vi "rotate.vi"(0 "Angle":dbl, 1 "Rate":dbl=-4.0) -> (2 "finished?":bool, 3 "left speed":dbl, 4 "right speed":dbl)   [LabVIEW 2012]
doc: "Rotates the robot for a certain number of degrees at a certain rate."
uses:
  <vilib>/addons/control/pid/pid.llb/PID Control Input Filter (DBL).vi
  <vilib>/addons/control/pid/NI_PID_pid.lvlib
  <vilib>/addons/control/pid/pid.llb/PID (DBL).vi
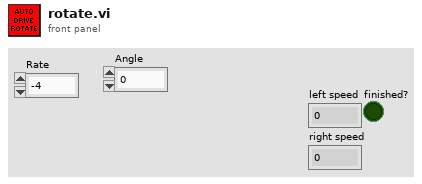
[diagram p1: front panel]
types:
  T1 = typedef "subStates.ctl" = enum16{"null", "wait", "driver control", "auto", "manual override", "hold position", "rotate", "feeder", "end"}
  T2 = typedef "WPI_EncoderDevRef.ctl" = cluster{"DevStatus":errorcluster, "EncoderIndex":T3, "CounterIndex":T4, "DistancePerCount":dbl, "Decoding Type":T5}
  T3 = typedef "FPGA_EncoderIdx.ctl" = enum8{"Enc 0", "Enc 1", "Enc 2", "Enc 3", "Invalid"}
  T4 = typedef "FPGA_CounterCtrSystemIndex.ctl" = enum8{"Ctr 0", "Ctr 1", "Ctr 2", "Ctr 3", "Ctr 4", "Ctr 5", "Ctr 6", "Ctr 7", "Invalid"}
  T5 = typedef "WPI_EncoderType.ctl" = enum16{"1x", "2x", "4x"}
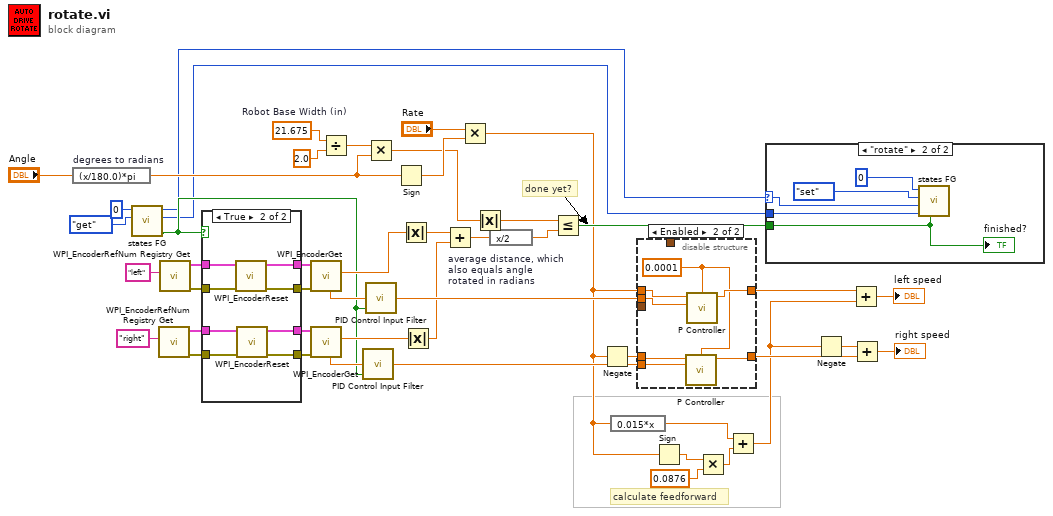
[diagram p0: block diagram]
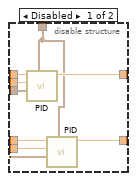
[diagram p2: hidden frame]
diagram:
  w46 = 21.675  # Robot Base Width (in)
  # "calculate feedforward"
  # "done yet?"
  n1 = expression code="(x/180.0)*pi" "degrees to radians"("Angle") -> (w4:dbl)
  n2 = call "states FG.vi"("menu (get)"=enum16{"set", "get"}."get", "Loop ID"=0) -> ("first call?"=w19:bool, "state # out"=w2:i32, "subState out"=w1:T1)  [unwired: 6 in, 1 out]
  n3 = call <vilib>:"WPI_EncoderRefNum Registry Get.vi"("refnum name"="right") -> ("error out"=w30:errorcluster, "EncoderDevRef"=w31:T2)  [unwired: 9 in]
  n4 = call <vilib>:"WPI_EncoderRefNum Registry Get.vi"("refnum name"="left") -> ("error out"=w32:errorcluster, "EncoderDevRef"=w33:T2)  [unwired: 9 in]
  n5 = case shown="True" w19 {
    tunnel: w33 -> [w51 w57]
    tunnel: w32 -> [w50 w59]
    tunnel: w31 -> [w49 w54]
    tunnel: w30 -> [w48 w55]
    tunnel: [w50 w58] -> w29
    tunnel: [w51 w56] -> w28
    tunnel: [w49 w53] -> w27
    tunnel: [w48 w52] -> w26
    frame False {
    }
    frame True {
      n6 = call <vilib>:"WPI_EncoderReset.vi"("error in (no error)"=w59, "EncoderDevRef"=w57) -> ("error out"=w58:errorcluster, "EncoderDevRef"=w56:T2)  [unwired: 8 in]
      n7 = call <vilib>:"WPI_EncoderReset.vi"("error in (no error)"=w55, "EncoderDevRef"=w54) -> ("error out"=w52:errorcluster, "EncoderDevRef"=w53:T2)  [unwired: 8 in]
    }
  }
  n8 = call <vilib>:"WPI_EncoderGet.vi"("error in (no error)"=w29, "EncoderDevRef"=w28) -> ("Distance"=w25:dbl, "Rate"=w38:dbl)  [unwired: 4 in, 4 out]
  n9 = call <vilib>:"WPI_EncoderGet.vi"("error in (no error)"=w26, "EncoderDevRef"=w27) -> ("Distance"=w24:dbl, "Rate"=w37:dbl)  [unwired: 4 in, 4 out]
  n10 = Divide(x=w46, y=2.0) -> (x/y=w45:dbl)
  n11 = call-poly <vilib>:"PID Control Input Filter.vi"("reinitialize? (F)"=w19, "input"=w37) -> ("output"=w20:dbl)  [unwired: 3 in]
  n12 = Multiply(x=w45, y=w4) -> (x*y=w16:dbl)
  n13 = call-poly <vilib>:"PID Control Input Filter.vi"("reinitialize? (F)"=w19, "input"=w38) -> ("output"=w21:dbl)  [unwired: 3 in]
  n14 = Sign(1:w4) -> (0:w17:dbl)
  n15 = Absolute Value(x=w25) -> (abs(x)=w15:dbl)
  n16 = Absolute Value(x=w24) -> (abs(x)=w14:dbl)
  n17 = Add(x=w15, y=w14) -> (x+y=w36:dbl)
  n18 = Multiply(x="Rate", y=w17) -> (x*y=w10:dbl)
  n19 = Absolute Value(x=w16) -> (abs(x)=w3:dbl)
  n20 = expression code="x/2" "average distance, which also equals angle rotated in radians"(w36) -> (w35:dbl)
  n21 = Less Or Equal?(x=w3, y=w35) -> (x <= y?=w34:bool)
  n22 = Negate(x=w10) -> (-x=w13:dbl)
  n23 = expression code="0.015*x"(w10) -> (w8:dbl)
  n24 = disable-structure shown="Enabled" {
    disable-tunnel: [w67 w71] -> w44
    disable-tunnel: [w66 w72] -> w43
    disable-tunnel: _ -> [w65 _]
    disable-tunnel: w21 -> [w64 w73]
    disable-tunnel: w20 -> [w63 w69]
    disable-tunnel: _ -> [w62 _]
    disable-tunnel: w13 -> [w61 w70]
    disable-tunnel: w10 -> [w60 w74]
    frame Disabled {
      n25 = call-poly <vilib>:"PID.vi"("output range"=w65, "PID gains"=w62, "process variable"=w64, "setpoint"=w60) -> ("output"=w66:dbl)  [unwired: 6 in, 1 out]
      n26 = call-poly <vilib>:"PID.vi"("output range"=w65, "PID gains"=w62, "process variable"=w63, "setpoint"=w61) -> ("output"=w67:dbl)  [unwired: 6 in, 1 out]
    }
    frame Enabled {
      w68 = 0.0001 ("proportional gain (Kc)")
      n27 = call "P Controller.vi"("Kp"=w68, "Setpoint"=w70, "Process Variable"=w69) -> ("Output"=w71:dbl)  [unwired: 5 in]
      n28 = call "P Controller.vi"("Kp"=w68, "Setpoint"=w74, "Process Variable"=w73) -> ("Output"=w72:dbl)  [unwired: 5 in]
    }
  }
  n29 = Sign(1:w10) -> (0:w12:dbl)
  n30 = Multiply(x=w12, y=0.0876) -> (x*y=w9:dbl)
  n31 = Add(x=w8, y=w9) -> (x+y=w6:dbl)
  n32 = case shown="\"rotate\"" w1 {
    selector: w1 -> [_ w75]
    tunnel: w34 -> [_ w78]
    tunnel: w2 -> [_ w76]
    frame "null", Default {
    }
    frame "rotate" {
      n33 = call "states FG.vi"("exit in"=w78, "state # in"=w76, "subState in"=w75, "menu (get)"=enum16{"set", "get"}."set", "Loop ID"=0) -> ()  [unwired: 3 in, 4 out]
      "finished?" <- w78
    }
  }
  n34 = Negate(x=w6) -> (-x=w7:dbl)
  n35 = Add(x=w43, y=w6) -> (x+y=→"left speed":dbl)
  n36 = Add(x=w7, y=w44) -> (x+y=→"right speed":dbl)
